vi "initIxon.vi"() -> (5 "model":string, 6 "vsArray":dbl[](array[numeric]), 7 "hsArray":dbl[](array[numeric]))   [LabVIEW 2016]
uses:
  <userlib>/atmcd64d.llb/Error Code Enum typedef.ctl
  <userlib>/atmcd64d.llb/Shutter_type typedef.ctl
  <userlib>/atmcd64d.llb/FanMode_mode typedef.ctl
  <userlib>/atmcd64d.llb/Shutter_mode typedef.ctl
  <userlib>/atmcd64d.llb/ReadMode_mode typedef.ctl
  <userlib>/atmcd64d.llb/HSSpeed_type typedef.ctl
  <userlib>/atmcd64d.llb/AcquisitionMode_mode typedef.ctl
  <vilib>/Utility/miscctls.llb/LVStringsAndValuesArrayTypeDef_U16.ctl
  variables/imageSettings.vi
  variables/configDB.vi
panel:
  out "DLL error code from ini":u32
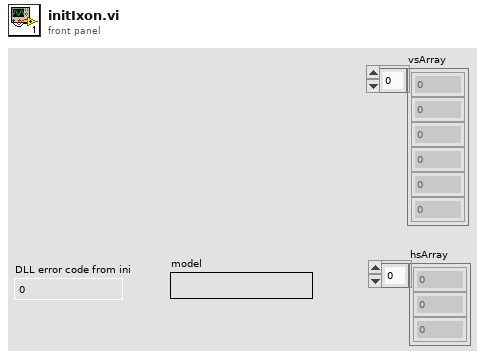
[diagram p1: front panel]
types:
  T1 = typedef "Error Code Enum typedef.ctl" = enum32{"N/A (0)", "DRV_ERROR_CODES", "DRV_SUCCESS", "DRV_VXDNOTINSTALLED", "DRV_ERROR_SCAN", "DRV_ERROR_CHECK_SUM", "DRV_ERROR_FILELOAD", "DRV_UNKNOWN_FUNC", "DRV_ERROR_VXD_INIT", "DRV_ERROR_ADDRESS", "DRV_ERROR_PAGELOCK", "DRV_ERROR_PAGEUNLOCK", "DRV_ERROR_BOARDTEST", "DRV_ERROR_ACK", "DRV_ERROR_UP_FIFO", "DRV_ERROR_PATTERN", "N/A (16)", "DRV_ACQUISITION_ERRORS", "DRV_ACQ_BUFFER", "DRV_ACQ_DOWNFIFO_FULL", "DRV_PROC_UNKONWN_INSTRUCTION", "DRV_ILLEGAL_OP_CODE", "DRV_KINETIC_TIME_NOT_MET", "DRV_ACCUM_TIME_NOT_MET", "DRV_NO_NEW_DATA", "N/A (25)", "DRV_SPOOLERROR", "N/A (27)", "N/A (28)", "N/A (29)", "N/A (30)", "N/A (31)", "N/A (32)", "DRV_TEMPERATURE_CODES", "DRV_TEMPERATURE_OFF", "DRV_TEMPERATURE_NOT_STABILIZED", "DRV_TEMPERATURE_STABILIZED", "DRV_TEMPERATURE_NOT_REACHED", "DRV_TEMPERATURE_OUT_RANGE", "DRV_TEMPERATURE_NOT_SUPPORTED", "DRV_TEMPERATURE_DRIFT", "N/A (41)", "N/A (42)", "N/A (43)", "N/A (44)", "N/A (45)", "N/A (46)", "N/A (47)", "N/A (48)", "DRV_GENERAL_ERRORS", "DRV_INVALID_AUX", "DRV_COF_NOTLOADED", "DRV_FPGAPROG", "DRV_FLEXERROR", "DRV_GPIBERROR", "N/A (55)", "N/A (56)", "N/A (57)", "N/A (58)", "N/A (59)", "N/A (60)", "N/A (61)", "N/A (62)", "N/A (63)", "DRV_DATATYPE", "DRV_DRIVER_ERRORS", "DRV_P1INVALID", "DRV_P2INVALID", "DRV_P3INVALID", "DRV_P4INVALID", "DRV_INIERROR", "DRV_COFERROR", "DRV_ACQUIRING", "DRV_IDLE", "DRV_TEMPCYCLE", "DRV_NOT_INITIALIZED", "DRV_P5INVALID", "DRV_P6INVALID", "DRV_INVALID_MODE", "DRV_INVALID_FILTER", "DRV_I2CERRORS", "DRV_I2CDEVNOTFOUND", "DRV_I2CTIMEOUT", "DRV_P7INVALID", "N/A (84)", "N/A (85)", "N/A (86)", "N/A (87)", "N/A (88)", "N/A (89)", "DRV_IOCERROR", "DRV_VRMVERSIONERROR"}
  T2 = typedef "Shutter_mode typedef.ctl" = enum16{"Auto", "Open", "Close", "N/A (3)", "Open FVB Series", "Open Any Series"}
  T3 = typedef "FanMode_mode typedef.ctl" = enum16{"fan on full", "fan on low", "fan off"}
  T4 = typedef "Shutter_type typedef.ctl" = enum16{"TTL Low", "TTL High"}
  T5 = typedef "LVStringsAndValuesArrayTypeDef_U16.ctl" = cluster{"String":string, "Value":u16}[]
  T6 = typedef "AcquisitionMode_mode typedef.ctl" = enum16{"Reserved (0)", "Single Scan", "Accumulate", "Kinetics", "Fast Kinetics", "Run Till Abort", "Reserved (6)", "Reserved (7)", "Reserved (8)", "Time Delayed Integration"}
  T7 = typedef "ReadMode_mode typedef.ctl" = enum16{"Full Vertical Binning", "Multi-Track", "Random-Track", "Single-Track", "Image"}
  T8 = typedef "HSSpeed_type typedef.ctl" = enum16{"EM Amp", "Conventional Amp"}
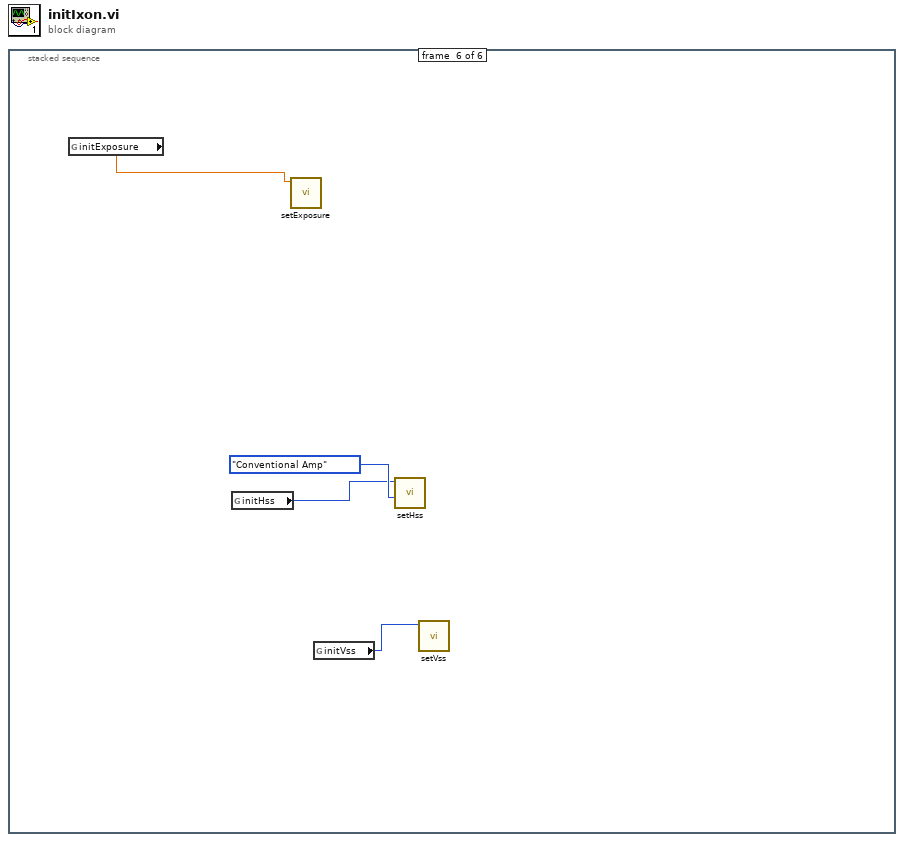
[diagram p0: block diagram]
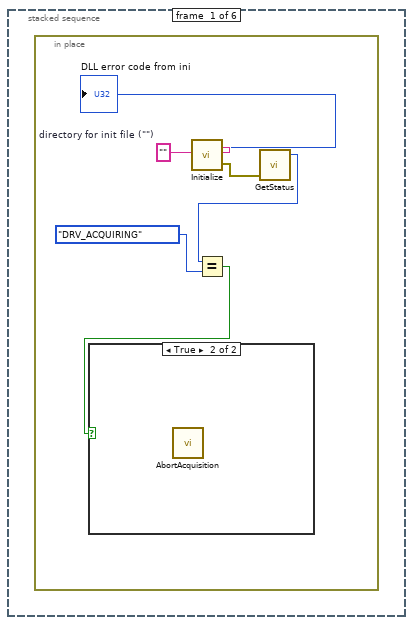
[diagram p2: hidden frame]
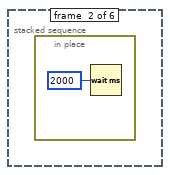
[diagram p4: hidden frame]
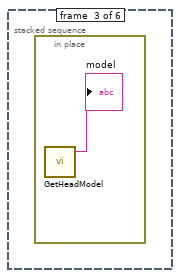
[diagram p5: hidden frame]
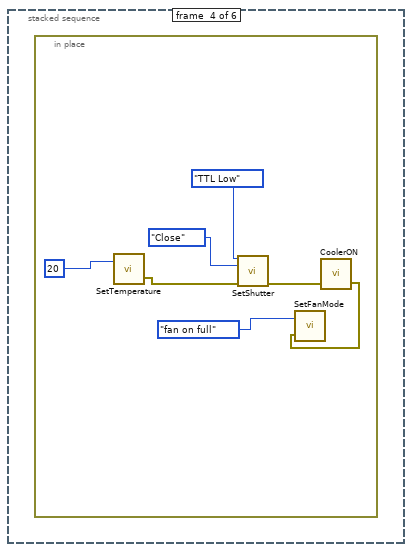
[diagram p6: hidden frame]
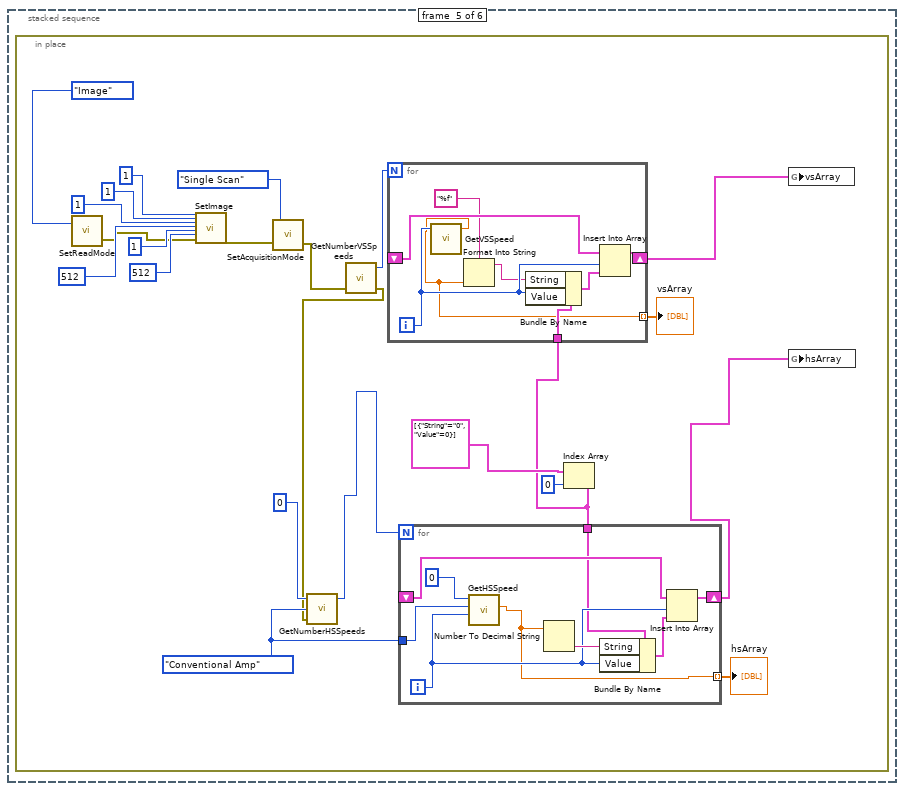
[diagram p7: hidden frame]
diagram:
  n1 = stacked-sequence {
    frame #0 {
      n2 = in-place {
        w6 = ""  # directory for init file ("")
        n3 = call <userlib>:"Initialize.vi"("directory (\"\")"=w6) -> ("error out"=w4:errorcluster, "DLL error code"=→"DLL error code from ini":u32)  [unwired: 1 in]
        n4 = call <userlib>:"GetStatus.vi"("error in (no error)"=w4) -> ("status"=w3:T1)  [unwired: 2 in, 2 out]
        n5 = Equal?(x=w3, y=Error_Code_Enum_typedef."DRV_ACQUIRING" ("status")) -> (x = y?=w1:bool)
        n6 = case shown="True" w1 {
          frame False {
          }
          frame True {
            n7 = call <userlib>:"AbortAcquisition.vi"() -> ()  [unwired: 2 in, 2 out]
          }
        }
      }
    }
    frame #1 {
      n8 = in-place {
        n9 = Wait (ms)(milliseconds to wait=u32 2000) -> ()  [unwired: 1 out]
      }
    }
    frame #2 {
      n10 = in-place {
        n11 = call <userlib>:"GetHeadModel.vi"() -> ("model"=→"model":string)  [unwired: 3 in, 2 out]
      }
    }
    frame #3 {
      n12 = in-place {
        n13 = call <userlib>:"SetTemperature.vi"("temperature"=20) -> ("error out"=w12:errorcluster)  [unwired: 1 in, 1 out]
        n14 = call <userlib>:"SetShutter.vi"("type"=Shutter_type_typedef."TTL Low", "mode"=Shutter_mode_typedef."Close", "error in (no error)"=w12) -> ("error out"=w13:errorcluster)  [unwired: 11 in, 1 out]
        n15 = call <userlib>:"CoolerON.vi"("error in (no error)"=w13) -> ("error out"=w10:errorcluster)  [unwired: 1 in, 1 out]
        n16 = call <userlib>:"SetFanMode.vi"("error in (no error)"=w10, "mode"=FanMode_mode_typedef."fan on full") -> ()  [unwired: 2 out]
      }
    }
    frame #4 {
      n17 = in-place {
        w28 = HSSpeed_type_typedef."Conventional Amp" ("type")
        n18 = call <userlib>:"SetReadMode.vi"("mode"=ReadMode_mode_typedef."Image") -> ("error out"=w31:errorcluster)  [unwired: 1 in, 1 out]
        n19 = call <userlib>:"SetImage.vi"("hbin"=1, "vbin"=1, "hstart"=1, "hend"=512, "vstart"=1, "vend"=512, "error in (no error)"=w31) -> ("error out"=w25:errorcluster)  [unwired: 19 in, 1 out]
        n20 = call <userlib>:"SetAcquisitionMode.vi"("error in (no error)"=w25, "mode"=AcquisitionMode_mode_typedef."Single Scan") -> ("error out"=w24:errorcluster)  [unwired: 1 out]
        n21 = call <userlib>:"GetNumberVSSpeeds.vi"("error in (no error)"=w24) -> ("error out"=w26:errorcluster, "number"=w30:i32)  [unwired: 2 in, 1 out]
        n22 = call <userlib>:"GetNumberHSSpeeds.vi"("error in (no error)"=w26, "type"=w28, "channel"=0) -> ("number"=w27:i32)  [unwired: 2 out]
        n23 = Index Array(array=T5 [{"String"="0", "Value"=0}] ("Strings And Values []"), index=0) -> (element=w20:cluster{"String":string, "Value":u16})
        n24 = for {
          N: w30 -> [_]
          tunnel: w20 -> [w55]
          shift-right: [w52] -> w19
          shift-left: _ -> [w51]
          tunnel: [w48] -> w17 mode=indexing
          i -> [w53]
          n25 = call <userlib>:"GetVSSpeed.vi"("index"=w53) -> ("speed"=w48:sgl)  [unwired: 2 in, 2 out]
          n26 = Format Into String(format string="%f", w48) -> (resulting string=w50:string)  [unwired: 2 in, 1 out]
          n27 = Bundle By Name(cluster=w55, "String"=w50, "Value"=w53) -> (w54:cluster{"String":string, "Value":u16})
          n28 = Insert Into Array(array=w51, index=w53, new element=w54) -> (w52:cluster{"String":string, "Value":u16}[])
        }
        "vsArray" <- w17
        n29 = for {
          N: w27 -> [_]
          tunnel: w28 -> [w46]
          shift-right: [w42] -> w18
          shift-left: _ -> [w41]
          tunnel: w20 -> [w40]
          tunnel: [w39] -> w16 mode=indexing
          i -> [w43]
          n30 = call <userlib>:"GetHSSpeed.vi"("index"=w43, "type"=w46, "channel"=0) -> ("speed"=w39:sgl)  [unwired: 2 in, 2 out]
          n31 = Number To Decimal String(number=w39) -> (decimal integer string=w45:string)  [unwired: 1 in]
          n32 = Bundle By Name(cluster=w40, "String"=w45, "Value"=w43) -> (w44:cluster{"String":string, "Value":u16})
          n33 = Insert Into Array(array=w41, index=w43, new element=w44) -> (w42:cluster{"String":string, "Value":u16}[])
        }
        "hsArray" <- w16
        n34 = global write "imageSettings.vi" "vsArray"(w19) -> ()
        n35 = global write "imageSettings.vi" "hsArray"(w18) -> ()
      }
    }
    frame #5 {
      n36 = global read "configDB.vi" "initExposure"() -> (w59:dbl)
      n37 = global read "configDB.vi" "initHss"() -> (w57:i32)
      n38 = call "setExposure.vi"("Exposure Time (s)"=w59) -> ()  [unwired: 11 in]
      n39 = global read "configDB.vi" "initVss"() -> (w56:i32)
      n40 = call "setHss.vi"("type"=HSSpeed_type_typedef."Conventional Amp", "index"=w57) -> ()  [unwired: 10 in]
      n41 = call "setVss.vi"("index"=w56) -> ()  [unwired: 11 in]
    }
  }
